vi "Convert Variant to Dialog Options.vi"(8 "error in (no error)":errorcluster, 11 "dialog options variant":variant) -> (0 "error out":errorcluster, 3 "dialog options":T1={"angle mode"=1, "picture pixels per unit"=30.0, "close window on exit"=FALSE, "window behavior"=enum."Default"} {"angle mode" items=["Degrees", "Radians"]})   [LabVIEW 2017, in "NI_Robotics_Configure Steering Frame.lvlib"]
uses:
  <vilib>/robotics/Dialog/Configure Steering Frame/NI_Robotics_Configure Steering Frame.lvlib
  <vilib>/robotics/Dialog/Configure Steering Frame/Dialog Options.ctl
  <vilib>/robotics/Dialog/Configure Steering Frame/Angle Mode.ctl
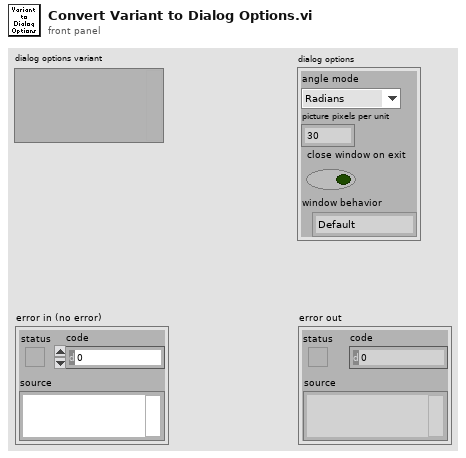
[diagram p1: front panel]
types:
  T1 = typedef "NI_Robotics_Configure Steering Frame.lvlib/Dialog Options.ctl" = cluster{"angle mode":T2, "picture pixels per unit":dbl, "close window on exit":bool, "window behavior":enum32{"Invalid", "Default", "Floating", "Floating/Auto-Hide", "Modal"}}
  T2 = typedef "NI_Robotics_Configure Steering Frame.lvlib/Angle Mode.ctl" = u16
  T3 = enum32{"Invalid", "Default", "Floating", "Floating/Auto-Hide", "Modal"}
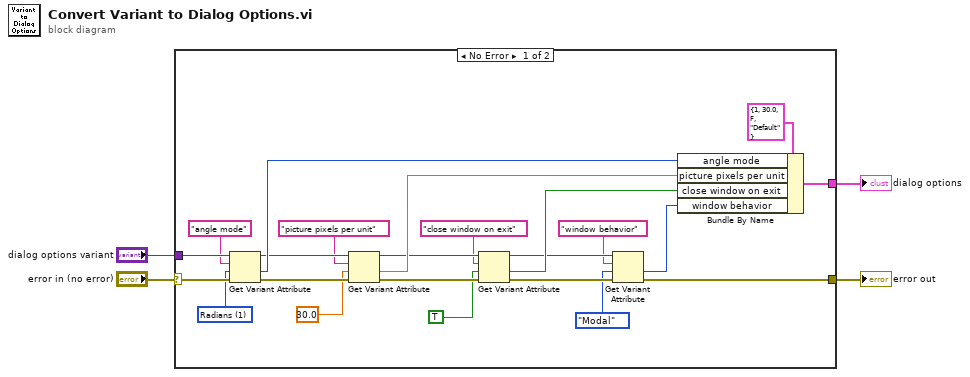
[diagram p0: block diagram]
diagram:
  n1 = case shown="No Error" "error in (no error)" {
    selector: "error in (no error)" -> [w26 w28]
    tunnel: [w7 w28] -> w3
    tunnel: "dialog options variant" -> [w27 _]
    tunnel: [w5 _] -> w1
    frame No Error {
      w23 = T2 1 items=["Degrees", "Radians"] ("angle mode")
      n2 = Get Variant Attribute(Variant=w27, name="angle mode", default value (empty Variant)=w23, error in=w26) -> (duplicate Variant=w21:variant, value=w22:T2, error out=w20:errorcluster)  [unwired: 1 out]
      n3 = Get Variant Attribute(Variant=w21, name="picture pixels per unit", default value (empty Variant)=30.0 ("picture pixels per unit"), error in=w20) -> (duplicate Variant=w16:variant, value=w17:dbl, error out=w14:errorcluster)  [unwired: 1 out]
      n4 = Get Variant Attribute(Variant=w16, name="close window on exit", default value (empty Variant)=TRUE ("close window on exit"), error in=w14) -> (duplicate Variant=w11:variant, value=w12:bool, error out=w9:errorcluster)  [unwired: 1 out]
      n5 = Get Variant Attribute(Variant=w11, name="window behavior", default value (empty Variant)=T3."Modal" ("window behavior"), error in=w9) -> (value=w6:T3, error out=w7:errorcluster)  [unwired: 2 out]
      n6 = Bundle By Name(cluster=T1 {"angle mode"=1, "picture pixels per unit"=30.0, "close window on exit"=FALSE, "window behavior"=enum."Default"} ("dialog options"), "angle mode"=w22, "picture pixels per unit"=w17, "close window on exit"=w12, "window behavior"=w6) -> (w5:T1)
    }
    frame Error {
    }
  }
  "error out" <- w3
  "dialog options" <- w1
